vi "ReadPanel.vi"(1 "reference":refnum<vi>) -> (0 "Panel":T4)   [LabVIEW 2013]
uses:
  <vilib>/Utility/miscctls.llb/LVBoundsTypeDef.ctl
  <vilib>/Utility/miscctls.llb/LVPositionTypeDef.ctl
  <vilib>/Utility/miscctls.llb/LVRectTypeDef.ctl
panel:
  out "error out 21":errorcluster
  out "error out 20":errorcluster
  out "error out 19":errorcluster
  out "error out 18":errorcluster
  out "error out 17":errorcluster
  out "error out 16":errorcluster
  out "error out 15":errorcluster
  out "error out 14":errorcluster
  out "error out 13":errorcluster
  out "error out 12":errorcluster
  out "error out 11":errorcluster
  out "error out 10":errorcluster
  out "error out 9":errorcluster
  out "error out 8":errorcluster
  out "error out 7":errorcluster
  out "error out 6":errorcluster
  out "error out 5":errorcluster
  out "error out 4":errorcluster
  out "error out 3":errorcluster
  out "error out 2":errorcluster
  out "error out":errorcluster
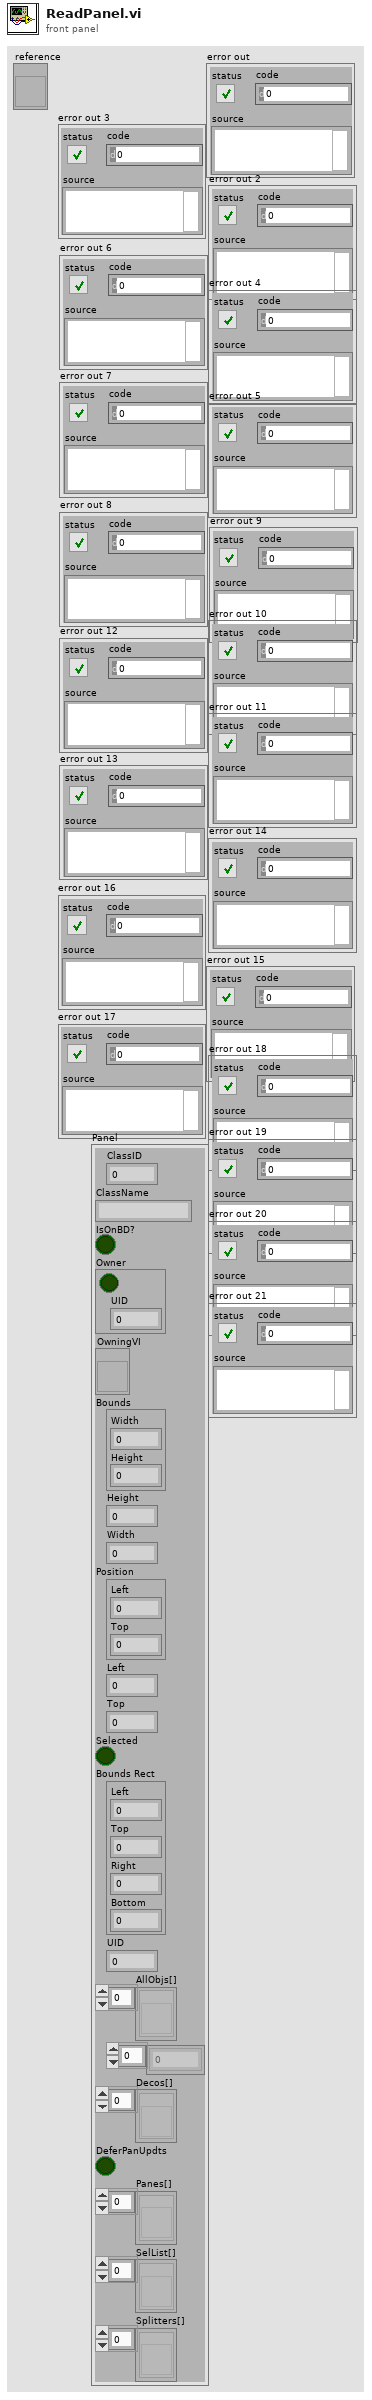
[diagram p1: front panel]
types:
  T1 = typedef "LVBoundsTypeDef.ctl" = cluster{"Width":u32, "Height":u32}
  T2 = typedef "LVPositionTypeDef.ctl" = cluster{"Left":i32, "Top":i32}
  T3 = typedef "LVRectTypeDef.ctl" = cluster{"Left":i16, "Top":i16, "Right":i16, "Bottom":i16}
  T4 = cluster{"ClassID":u32, "ClassName":string, "IsOnBD?":bool, "Owner":cluster{bool, "UID":i32}, "OwningVI":refnum<vi>, "Bounds":T1, "Height":u32, "Width":u32, "Position":T2, "Left":i32, "Top":i32, "Selected":bool, "Bounds Rect":T3, "UID":i32, "AllObjs[]":refnum<vi>[], "Controls[]":i32[], "Decos[]":refnum<vi>[], "DeferPanUpdts":bool, "Panes[]":refnum<vi>[], "SelList[]":refnum<vi>[], "Splitters[]":refnum<vi>[]}
  T5 = cluster{"ClassID":u32, "ClassName":string, "IsOnBD?":bool, "Cluster":cluster{bool, "UID":i32}, "OwningVI":refnum<vi>, "Bounds":T1, "Height":u32, "Width":u32, "Position":T2, "Left":i32, "Top":i32, "Selected":bool, "Bounds Rect":T3, "UID":i32, "AllObjs[]":refnum<vi>[], i32[], "Decos[]":refnum<vi>[], "DeferPanUpdts":bool, "Panes[]":refnum<vi>[], "SelList[]":refnum<vi>[], "Splitters[]":refnum<vi>[]}
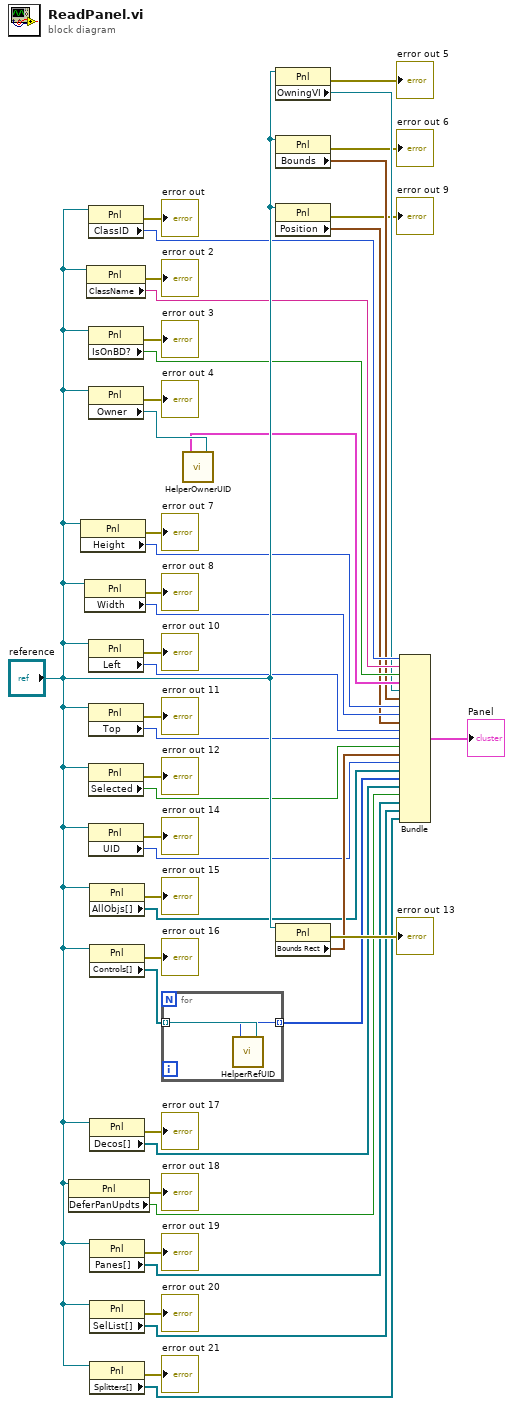
[diagram p0: block diagram]
diagram:
  n1 = property class="Pnl"(reference="reference") -> (error out=→"error out 18":errorcluster, "DeferPanUpdts"=w8:bool)  [unwired: 1 in, 1 out]
  n2 = property class="Pnl"(reference="reference") -> (error out=→"error out 7":errorcluster, "Height"=w31:u32)  [unwired: 1 in, 1 out]
  n3 = property class="Pnl"(reference="reference") -> (error out=→"error out 8":errorcluster, "Width"=w29:u32)  [unwired: 1 in, 1 out]
  n4 = property class="Pnl"(reference="reference") -> (error out=→"error out 2":errorcluster, "ClassName"=w42:string)  [unwired: 1 in, 1 out]
  n5 = property class="Pnl"(reference="reference") -> (error out=→"error out":errorcluster, "ClassID"=w44:u32)  [unwired: 1 in, 1 out]
  n6 = property class="Pnl"(reference="reference") -> (error out=→"error out 3":errorcluster, "IsOnBD?"=w40:bool)  [unwired: 1 in, 1 out]
  n7 = property class="Pnl"(reference="reference") -> (error out=→"error out 4":errorcluster, "Owner"=w38:refnum<vi>)  [unwired: 1 in, 1 out]
  n8 = property class="Pnl"(reference="reference") -> (error out=→"error out 10":errorcluster, "Left"=w25:i32)  [unwired: 1 in, 1 out]
  n9 = property class="Pnl"(reference="reference") -> (error out=→"error out 11":errorcluster, "Top"=w23:i32)  [unwired: 1 in, 1 out]
  n10 = property class="Pnl"(reference="reference") -> (error out=→"error out 12":errorcluster, "Selected"=w21:bool)  [unwired: 1 in, 1 out]
  n11 = property class="Pnl"(reference="reference") -> (error out=→"error out 14":errorcluster, "UID"=w17:i32)  [unwired: 1 in, 1 out]
  n12 = property class="Pnl"(reference="reference") -> (error out=→"error out 15":errorcluster, "AllObjs[]"=w15:refnum<vi>[])  [unwired: 1 in, 1 out]
  n13 = property class="Pnl"(reference="reference") -> (error out=→"error out 16":errorcluster, "Controls[]"=w13:refnum<vi>[])  [unwired: 1 in, 1 out]
  n14 = property class="Pnl"(reference="reference") -> (error out=→"error out 17":errorcluster, "Decos[]"=w10:refnum<vi>[])  [unwired: 1 in, 1 out]
  n15 = property class="Pnl"(reference="reference") -> (error out=→"error out 19":errorcluster, "Panes[]"=w6:refnum<vi>[])  [unwired: 1 in, 1 out]
  n16 = property class="Pnl"(reference="reference") -> (error out=→"error out 20":errorcluster, "SelList[]"=w4:refnum<vi>[])  [unwired: 1 in, 1 out]
  n17 = property class="Pnl"(reference="reference") -> (error out=→"error out 21":errorcluster, "Splitters[]"=w2:refnum<vi>[])  [unwired: 1 in, 1 out]
  n18 = for {
    tunnel: w13 -> [w48] mode=indexing
    tunnel: [w47] -> w12 mode=indexing
    n19 = call "HelperRefUID.vi"("Text in"=w48) -> ("UID"=w47:i32)
  }
  n20 = call "HelperOwnerUID.vi"("Generic in"=w38) -> ("Cluster"=w37:cluster{bool, "UID":i32})
  n21 = property class="Pnl"(reference="reference") -> (error out=→"error out 5":errorcluster, "OwningVI"=w35:refnum<vi>)  [unwired: 1 in, 1 out]
  n22 = property class="Pnl"(reference="reference") -> (error out=→"error out 6":errorcluster, "Bounds"=w33:T1)  [unwired: 1 in, 1 out]
  n23 = property class="Pnl"(reference="reference") -> (error out=→"error out 9":errorcluster, "Position"=w27:T2)  [unwired: 1 in, 1 out]
  n24 = property class="Pnl"(reference="reference") -> (error out=→"error out 13":errorcluster, "Bounds Rect"=w19:T3)  [unwired: 1 in, 1 out]
  n25 = Bundle("ClassID"=w44, "ClassName"=w42, "IsOnBD?"=w40, "Cluster"=w37, "OwningVI"=w35, "Bounds"=w33, "Height"=w31, "Width"=w29, "Position"=w27, "Left"=w25, "Top"=w23, "Selected"=w21, "Bounds Rect"=w19, "UID"=w17, "AllObjs[]"=w15, w12, "Decos[]"=w10, "DeferPanUpdts"=w8, "Panes[]"=w6, "SelList[]"=w4, "Splitters[]"=w2) -> (→"Panel":T5)  [unwired: 1 in]
